vi "ExSubSetInitCamSame.vi"(0 "Camera Handle":u32, 1 "Exposure":dbl min=0.0 step=0.001 format="%.3f", 3 "error in (no error)":errorcluster, 4 "Name":string) -> (5 "Handles Out":T1, 6 "error out":errorcluster)   [LabVIEW 2010]
panel:
  # "ExSubSetInitCam:\nThis sub vi initializes the camera."
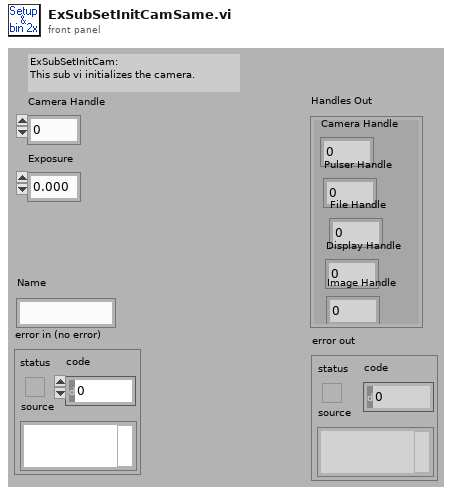
[diagram p1: front panel]
types:
  T1 = cluster{"Camera Handle":u32, "Pulser Handle":u32, "File Handle":u32, "Display Handle":u32, "Image Handle":u32}
  T2 = cluster{"acquire focus mode":u32, "Exposure":dbl, "Number of Images":u32, "Software accumulation":u32}
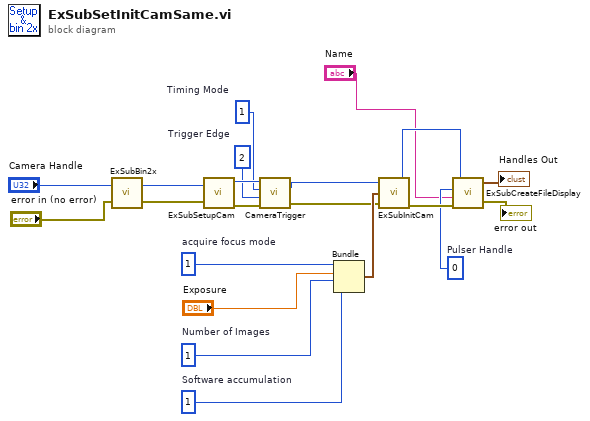
[diagram p0: block diagram]
diagram:
  w11 = u32 0  # Pulser Handle
  w12 = u32 1  # Timing Mode
  w13 = u32 2  # Trigger Edge
  w16 = u32 1  # acquire focus mode
  w15 = u32 1  # Number of Images
  w14 = u32 1  # Software accumulation
  n1 = call "ExSubBin2x.vi"("error in (no error)"="error in (no error)", "Camera Handle"="Camera Handle") -> ("error out"=w1:errorcluster, "Camera Handle"=w2:u32)
  n2 = call "ExSubSetupCam.vi"("error in (no error)"=w1, "Camera Handle"=w2) -> ("error out"=w17:errorcluster, "Camera Handle"=w18:u32)
  n3 = call <userlib>:"CameraTrigger.vi"("error in"=w17, "Trigger Edge"=w13, "Timing Mode"=w12, "Camera Handle"=w18) -> ("error out"=w3:errorcluster, "Camera Handle"=w4:u32)
  n4 = Bundle("acquire focus mode"=w16, "Exposure"="Exposure", "Number of Images"=w15, "Software accumulation"=w14) -> (w20:T2)  [unwired: 1 in]
  n5 = call "ExSubInitCam.vi"("error in (no error)"=w3, "Camera Information"=w20, "Camera Handle"=w4) -> ("error out"=w19:errorcluster, "Camera Handle"=w7:u32)
  n6 = call "ExSubCreateFileDisplay.vi"("error in (no error)"=w19, "File and Display Name"="Name", "Pulser Handle"=w11, "Camera Handle"=w7) -> ("error out"=→"error out":errorcluster, "Handles Out"=→"Handles Out":T1)
